vi "LoadLevel.vi"(8 "error in (no error)":errorcluster, 10 "Restart? (F)":bool, 11 "Game in":refnum<class "Game.lvclass">) -> (0 "error out":errorcluster, 3 "Game out":refnum<class "Game.lvclass">)   [LabVIEW 2019, in "RT_Game.lvlib" / "Game.lvclass"]
uses:
  Game.lvclass
  Menu/Menu.lvclass
  C:/Users/FreshBob/Dropbox/VIs/myRIO_GameConsole/RT/RT_Game/Game/Game.lvclass
  Game.lvclass/Game.ctl
  Read SlideInDirection.vi
  Write SlideInDirection.vi
  Write SwitchGame.vi
  Write FlattenedNextClass.vi
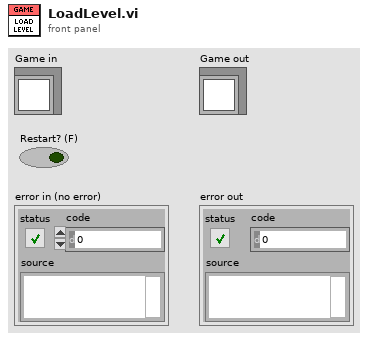
[diagram p1: front panel]
types:
  T1 = typedef "RT_Game.lvlib/Game.lvclass/ScreenSide.ctl" = enum16{"up", "down", "left", "right"}
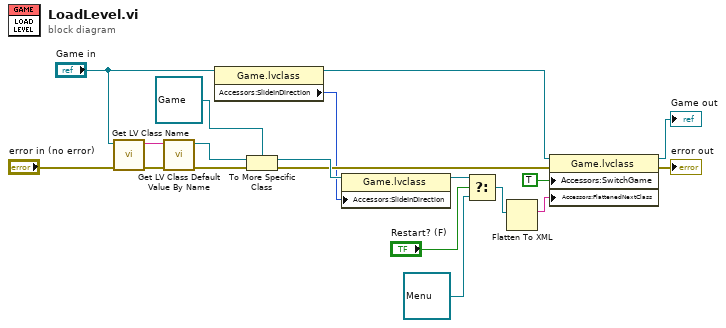
[diagram p0: block diagram]
diagram:
  n1 = call <vilib>:"Get LV Class Name.vi"("error in (no error)"="error in (no error)", "object"="Game in") -> ("error out"=w11:errorcluster, "class name"=w13:string)  [unwired: 8 in]
  n2 = call <vilib>:"Get LV Class Default Value By Name.vi"("error in (no error)"=w11, "class name"=w13) -> ("error out"=w12:errorcluster, "object"=w15:refnum<class>)  [unwired: 8 in]
  n3 = property class="Game.lvclass"(reference="Game in") -> (reference out=w2:refnum<class "Game.lvclass">, "Accessors:SlideInDirection"=w1:T1)  [unwired: 1 in, 1 out]
  n4 = To More Specific Class(target class=refnum<class "Game.lvclass"> refnum ("Game out"), reference=w15, error in=w12) -> (specific class reference=w17:refnum<class "Game.lvclass">, error out=w14:errorcluster)
  n5 = property class="Game.lvclass"(reference=w17, "Accessors:SlideInDirection"=w1) -> (reference out=w3:refnum<class "Game.lvclass">)  [unwired: 1 in, 1 out]
  n6 = Select(t=w3, s="Restart? (F)", f=refnum<class "Menu.lvclass"> refnum ("RT_Game.lvlib:Menu.lvclass")) -> (s? t:f=w8:refnum<class "Game.lvclass">)
  n7 = Flatten To XML(anything=w8) -> (xml string=w7:string)
  n8 = property class="Game.lvclass"(reference=w2, error in=w14, "Accessors:SwitchGame"=TRUE ("SwitchGame_"), "Accessors:FlattenedNextClass"=w7) -> (reference out=→"Game out":refnum<class "Game.lvclass">, error out=→"error out":errorcluster)
